vi "tnksimulation.vi"() -> ()   [LabVIEW 2021]
panel:
  in  "stop":bool
  out "Tank":dbl(slide) scale=0.0..100.0
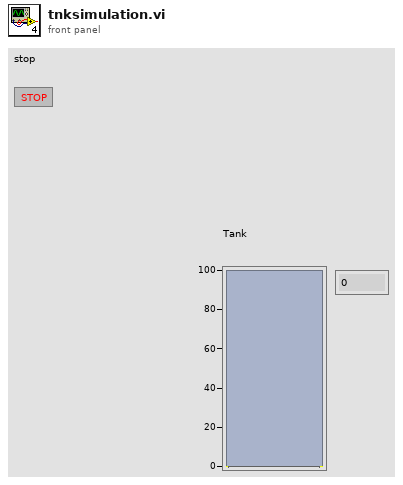
[diagram p1: front panel]
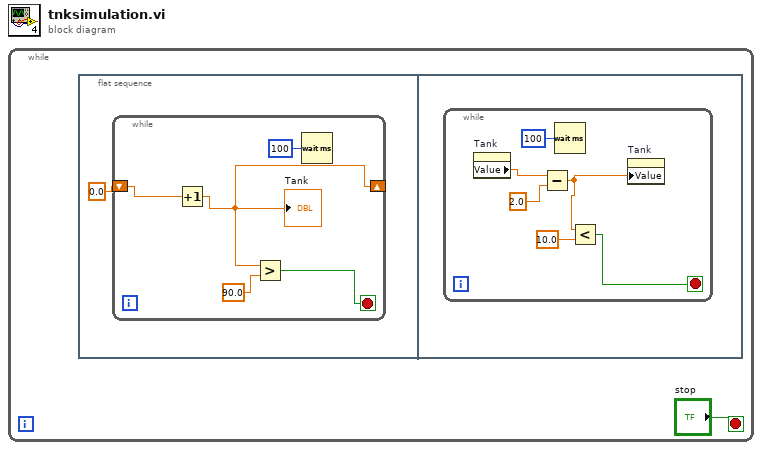
[diagram p0: block diagram]
diagram:
  n1 = while {
    stop <- "stop" stop-if-true
    n2 = flat-sequence {
      frame #0 {
        n3 = while {
          shift-right: [w6] -> _
          shift-left: 0.0 -> [w7]
          stop <- w4 stop-if-true
          n4 = Increment(x=w7) -> (x+1=w6:dbl)
          "Tank" <- w6
          n5 = Greater?(x=w6, y=90.0) -> (0:w4:bool)
          n6 = Wait (ms)(milliseconds to wait=u32 100) -> ()  [unwired: 1 out]
        }
      }
      frame #1 {
        n7 = while {
          stop <- w9 stop-if-true
          n8 = property on="Tank" class="Slide (strict)"() -> ("Value"=w13:dbl)  [unwired: 2 in, 2 out]
          n9 = Subtract(x=w13, y=2.0) -> (x-y=w11:dbl)
          n10 = Wait (ms)(milliseconds to wait=u32 100) -> ()  [unwired: 1 out]
          n11 = Less?(x=w11, y=10.0) -> (x < y?=w9:bool)
          n12 = property on="Tank" class="Slide (strict)"("Value"=w11) -> ()  [unwired: 2 in, 2 out]
        }
      }
    }
  }
